vi "speed control setting.vi"() -> ()   [LabVIEW 2019]
uses:
  database.lvlib
panel:
  in  "bias 6":dbl=14.0
  in  "bias 5":dbl=14.0
  in  "bias 4":dbl=6.0
  in  "bias 3":dbl=2.0
  in  "bias 2":dbl=6.0
  in  "bias 1":dbl=12.0 caption="Set Point"
  in  "Disc 06":dbl=12.0 min=11.0 max=13.0 step=0.1
  in  "Error in 2":errorcluster
  out "Error out":errorcluster
  in  "Error THR":dbl=1.5 caption="Max. Speed (RPM)" min=0.5 max=3.0 step=0.25
  in  "Close":bool
  in  "Max. Speed (RPM)":dbl=7.5 min=5.0 max=6.0 step=0.1
  in  "Min. Speed (RPM)":dbl=5.5 min=3.0 max=4.0 step=0.1
  in  "pulse period (sec)":dbl=240.0 caption="Speed Control" min=60.0 max=600.0
  in  "Disc 05":dbl=12.0 min=11.0 max=13.0 step=0.1
  in  "Disc 04":dbl=12.0 min=11.0 max=13.0 step=0.1
  in  "Disc 03":dbl=12.0 min=11.0 max=13.0 step=0.1
  in  "Disc 02":dbl=12.0 min=11.0 max=13.0 step=0.1
  in  "Disc 01":dbl=12.0 caption="Set Point" min=10.0 max=13.0 step=0.1
  out "Name":string="Control Setting"
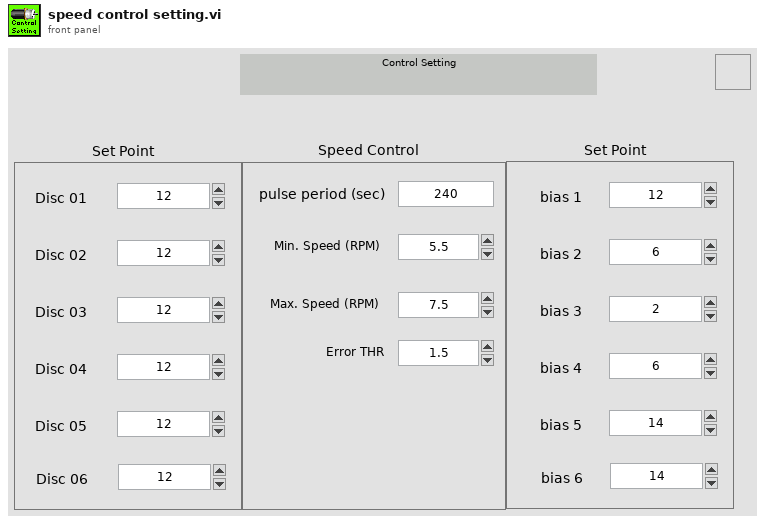
[diagram p1: front panel]
types:
  T1 = cluster{"Disc 01":dbl, "Disc 02":dbl, "Disc 03":dbl, "Disc 04":dbl, "Disc 05":dbl, "Disc 06":dbl, "pulse period (sec)":dbl, "Max. Speed (RPM)":dbl, "Min. Speed (RPM)":dbl, "Error THR":dbl, "bias 1":dbl, "bias 2":dbl, "bias 3":dbl, "bias 4":dbl, "bias 5":dbl, "bias 6":dbl}
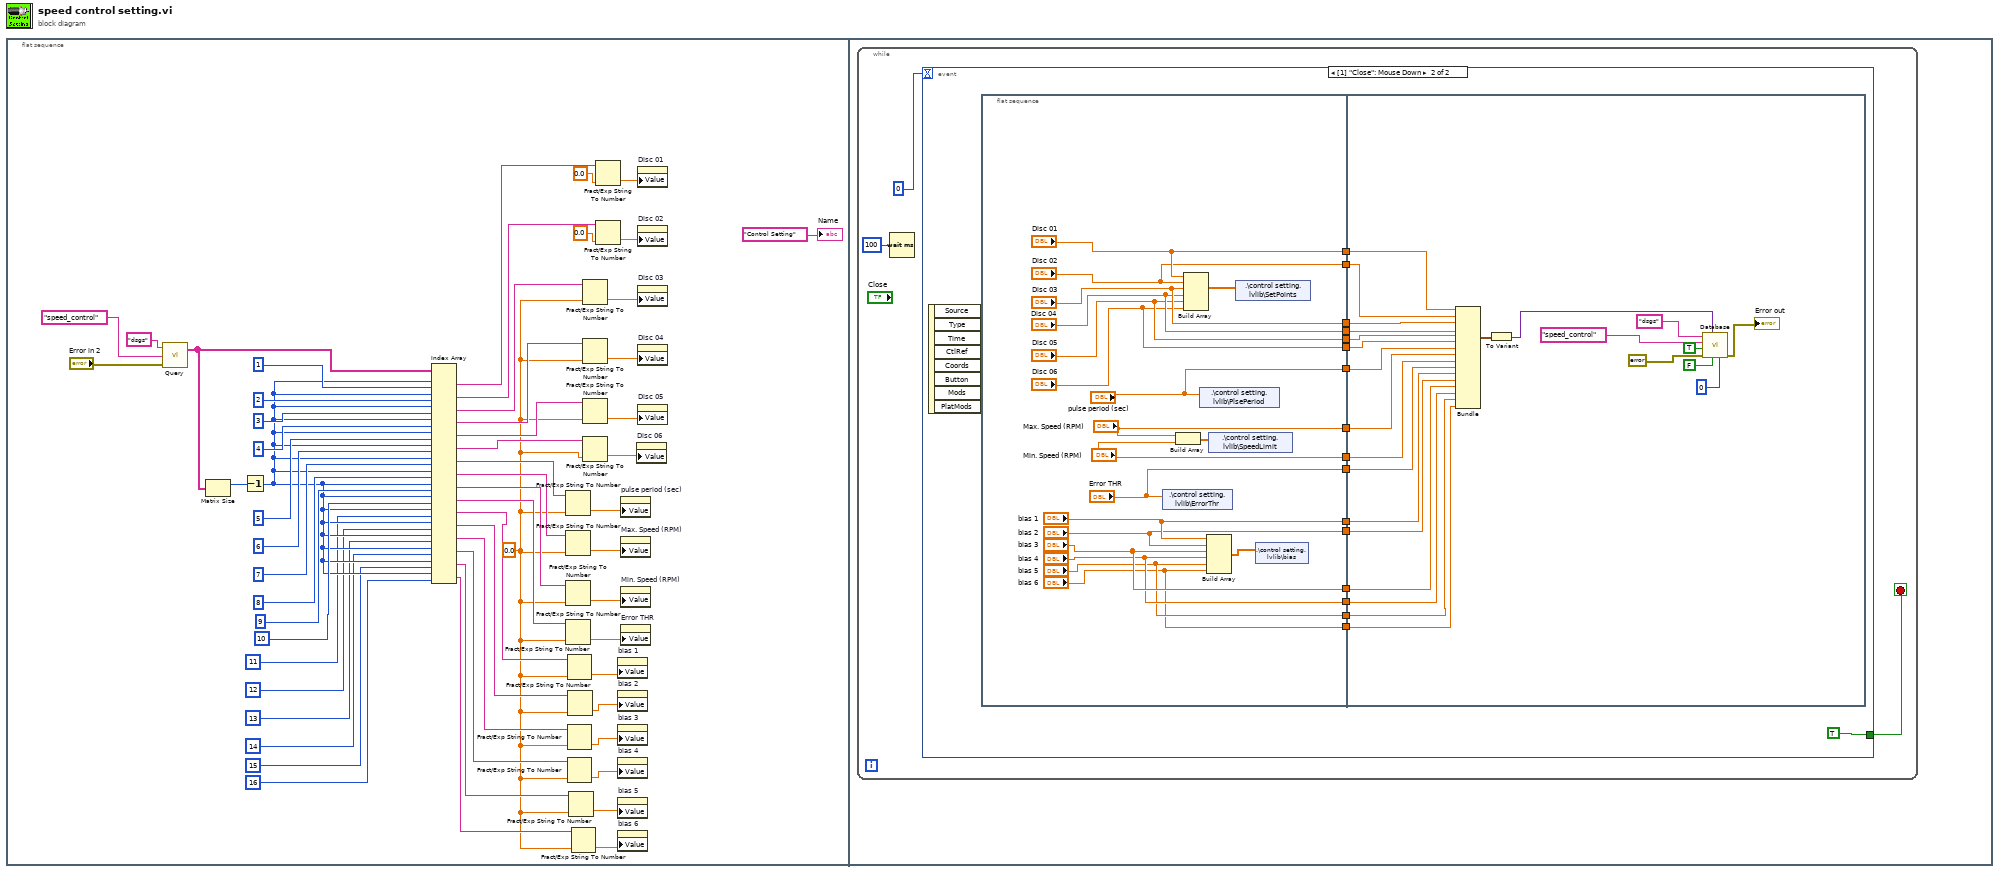
[diagram p0: block diagram]
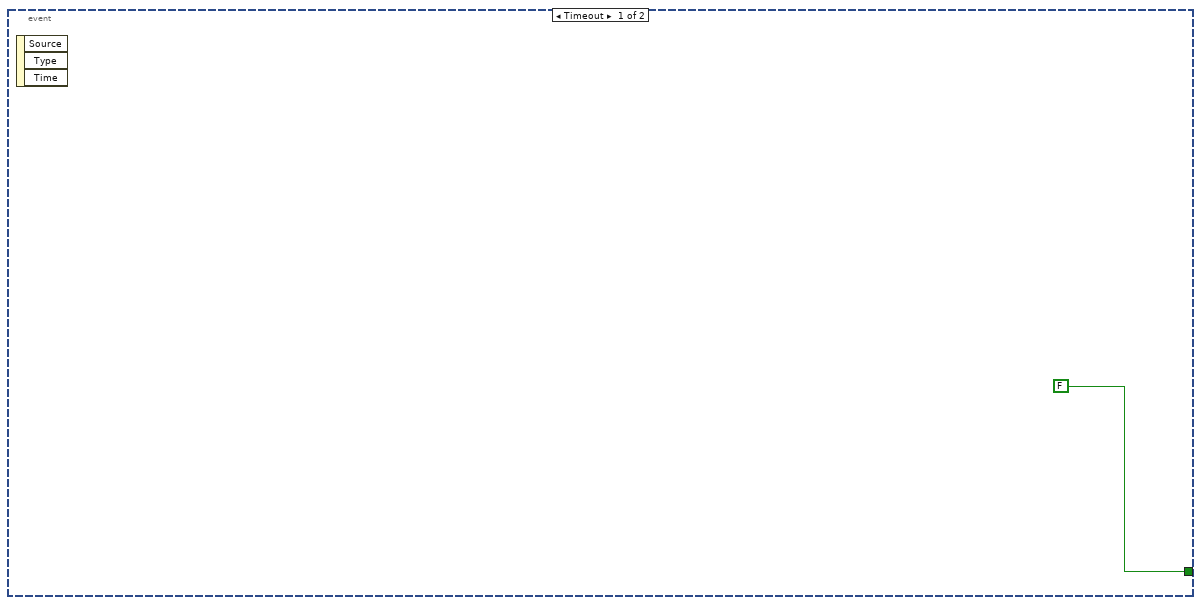
[diagram p2: hidden frame]
diagram:
  n1 = flat-sequence {
    frame #0 {
      w7 = 0.0 ("default (0 DBL)")
      n2 = call "Query.vi"("Error in"="Error in 2", "Table Name"="speed_control", "Connection Name"="dsgs") -> ("data"=w36:string[][])  [unwired: 1 in, 1 out]
      n3 = Matrix Size(0:w36) -> (1:w54:i32)  [unwired: 1 out]
      n4 = Decrement(x=w54) -> (x-1=w19:i32)
      n5 = Index Array(array=w36, index (row) #1=w19, index (col) #1=1 ("disabled index (col)"), index (row) #2=w19, index (col) #2=2 ("disabled index (col)"), index (row) #3=w19, index (col) #3=3 ("disabled index (col)"), index (row) #4=w19, index (col) #4=4 ("disabled index (col)"), index (row) #5=w19, index (col) #5=5 ("disabled index (col)"), index (row) #6=w19, index (col) #6=6 ("disabled index (col)"), index (row) #7=w19, index (col) #7=7 ("disabled index (col)"), index (row) #8=w19, index (col) #8=8 ("disabled index (col)"), index (row) #9=w19, index (col) #9=9 ("disabled index (col)"), index (row) #10=w19, index (col) #10=10 ("disabled index (col)"), index (row) #11=w19, index (col) #11=11 ("disabled index (col)"), index (row) #12=w19, index (col) #12=12 ("disabled index (col)"), index (row) #13=w19, index (col) #13=13 ("disabled index (col)"), index (row) #14=w19, index (col) #14=14 ("disabled index (col)"), index (row) #15=w19, index (col) #15=15 ("disabled index (col)"), index (row) #16=w19, index (col) #16=16 ("disabled index (col)")) -> (element #1=w44:string, element #2=w40:string, element #3=w39:string, element #4=w38:string, element #5=w37:string, element #6=w23:string, element #7=w24:string, element #8=w25:string, element #9=w26:string, element #10=w27:string, element #11=w20:string, element #12=w12:string, element #13=w11:string, element #14=w10:string, element #15=w9:string, element #16=w8:string)
      n6 = Fract/Exp String To Number(string=w24, default (0 dbl)=w7) -> (number=w31:dbl)  [unwired: 2 in, 1 out]
      n7 = Fract/Exp String To Number(string=w25, default (0 dbl)=w7) -> (number=w30:dbl)  [unwired: 2 in, 1 out]
      n8 = Fract/Exp String To Number(string=w26, default (0 dbl)=w7) -> (number=w29:dbl)  [unwired: 2 in, 1 out]
      n9 = Fract/Exp String To Number(string=w27, default (0 dbl)=w7) -> (number=w28:dbl)  [unwired: 2 in, 1 out]
      n10 = Fract/Exp String To Number(string=w20, default (0 dbl)=w7) -> (number=w6:dbl)  [unwired: 2 in, 1 out]
      n11 = Fract/Exp String To Number(string=w11, default (0 dbl)=w7) -> (number=w4:dbl)  [unwired: 2 in, 1 out]
      n12 = Fract/Exp String To Number(string=w10, default (0 dbl)=w7) -> (number=w3:dbl)  [unwired: 2 in, 1 out]
      n13 = Fract/Exp String To Number(string=w12, default (0 dbl)=w7) -> (number=w5:dbl)  [unwired: 2 in, 1 out]
      n14 = Fract/Exp String To Number(string=w9, default (0 dbl)=w7) -> (number=w2:dbl)  [unwired: 2 in, 1 out]
      n15 = Fract/Exp String To Number(string=w8, default (0 dbl)=w7) -> (number=w1:dbl)  [unwired: 2 in, 1 out]
      n16 = Fract/Exp String To Number(string=w39, default (0 dbl)=w7) -> (number=w34:dbl)  [unwired: 2 in, 1 out]
      n17 = Fract/Exp String To Number(string=w38, default (0 dbl)=w7) -> (number=w33:dbl)  [unwired: 2 in, 1 out]
      n18 = Fract/Exp String To Number(string=w37, default (0 dbl)=w7) -> (number=w32:dbl)  [unwired: 2 in, 1 out]
      n19 = Fract/Exp String To Number(string=w23, default (0 dbl)=w7) -> (number=w22:dbl)  [unwired: 2 in, 1 out]
      n20 = Fract/Exp String To Number(string=w44, default (0 dbl)=0.0 ("default (0 DBL)")) -> (number=w42:dbl)  [unwired: 2 in, 1 out]
      n21 = Fract/Exp String To Number(string=w40, default (0 dbl)=0.0 ("default (0 DBL)")) -> (number=w35:dbl)  [unwired: 2 in, 1 out]
      n22 = property on="bias 1" class="DigNum (strict)"("Value"=w6) -> ()  [unwired: 2 in, 2 out]
      n23 = property on="bias 2" class="DigNum (strict)"("Value"=w5) -> ()  [unwired: 2 in, 2 out]
      n24 = property on="bias 3" class="DigNum (strict)"("Value"=w4) -> ()  [unwired: 2 in, 2 out]
      n25 = property on="bias 4" class="DigNum (strict)"("Value"=w3) -> ()  [unwired: 2 in, 2 out]
      n26 = property on="bias 5" class="DigNum (strict)"("Value"=w2) -> ()  [unwired: 2 in, 2 out]
      n27 = property on="bias 6" class="DigNum (strict)"("Value"=w1) -> ()  [unwired: 2 in, 2 out]
      n28 = property on="pulse period (sec)" class="DigNum (strict)"("Value"=w31) -> ()  [unwired: 2 in, 2 out]
      n29 = property on="Max. Speed (RPM)" class="DigNum (strict)"("Value"=w30) -> ()  [unwired: 2 in, 2 out]
      n30 = property on="Min. Speed (RPM)" class="DigNum (strict)"("Value"=w29) -> ()  [unwired: 2 in, 2 out]
      n31 = property on="Error THR" class="DigNum (strict)"("Value"=w28) -> ()  [unwired: 2 in, 2 out]
      n32 = property on="Disc 06" class="DigNum (strict)"("Value"=w22) -> ()  [unwired: 2 in, 2 out]
      n33 = property on="Disc 01" class="DigNum (strict)"("Value"=w42) -> ()  [unwired: 2 in, 2 out]
      n34 = property on="Disc 02" class="DigNum (strict)"("Value"=w35) -> ()  [unwired: 2 in, 2 out]
      n35 = property on="Disc 03" class="DigNum (strict)"("Value"=w34) -> ()  [unwired: 2 in, 2 out]
      n36 = property on="Disc 04" class="DigNum (strict)"("Value"=w33) -> ()  [unwired: 2 in, 2 out]
      n37 = property on="Disc 05" class="DigNum (strict)"("Value"=w32) -> ()  [unwired: 2 in, 2 out]
      "Name" <- "Control Setting" ("Name")
    }
    frame #1 {
      n38 = while {
        stop <- w60 stop-if-true
        n39 = Wait (ms)(milliseconds to wait=u32 100) -> ()  [unwired: 1 out]
        n40 = event shown="[1] \"Close\": Mouse Down" {
          selector: _ -> [_ _]
          dyn-events: _ -> [_ _]
          timeout: 0 -> [_ _]
          tunnel: [FALSE TRUE] -> w60
          event Timeout {
            n41 = event-data() -> ()  [unwired: 1 in, 3 out]
          }
          event "Close": Mouse Down {
            n42 = event-data() -> ()  [unwired: 1 in, 8 out]
            n43 = flat-sequence {
              tunnel: ["Disc 01"] -> w78
              tunnel: ["Disc 02"] -> w77
              tunnel: ["Disc 03"] -> w76
              tunnel: ["Disc 04"] -> w75
              tunnel: ["Disc 05"] -> w74
              tunnel: ["pulse period (sec)"] -> w73
              tunnel: ["Max. Speed (RPM)"] -> w72
              tunnel: ["Min. Speed (RPM)"] -> w71
              tunnel: ["Error THR"] -> w70
              tunnel: ["Disc 06"] -> w69
              tunnel: ["bias 1"] -> w68
              tunnel: ["bias 2"] -> w67
              tunnel: ["bias 3"] -> w66
              tunnel: ["bias 4"] -> w65
              tunnel: ["bias 5"] -> w64
              tunnel: ["bias 6"] -> w63
              tunnel: w78 -> [w121]
              tunnel: w77 -> [w120]
              tunnel: w76 -> [w119]
              tunnel: w75 -> [w118]
              tunnel: w74 -> [w117]
              tunnel: w73 -> [w106]
              tunnel: w72 -> [w107]
              tunnel: w71 -> [w108]
              tunnel: w70 -> [w109]
              tunnel: w69 -> [w105]
              tunnel: w68 -> [w104]
              tunnel: w67 -> [w103]
              tunnel: w66 -> [w102]
              tunnel: w65 -> [w101]
              tunnel: w64 -> [w100]
              tunnel: w63 -> [w99]
              frame #0 {
                n44 = shared-variable ".\\control setting.lvlib\\ErrorThr"("Error THR") -> ()  [unwired: 1 in, 1 out]
                n45 = Build Array("Max. Speed (RPM)", "Min. Speed (RPM)") -> (w97:dbl[])
                n46 = Build Array("Disc 01", "Disc 02", "Disc 03", "Disc 04", "Disc 05", "Disc 06") -> (w98:dbl[])
                n47 = shared-variable ".\\control setting.lvlib\\PlsePeriod"("pulse period (sec)") -> ()  [unwired: 1 in, 1 out]
                n48 = Build Array("bias 1", "bias 2", "bias 3", "bias 4", "bias 5", "bias 6") -> (w86:dbl[])
                n49 = shared-variable ".\\control setting.lvlib\\SpeedLimit"(w97) -> ()  [unwired: 1 in, 1 out]
                n50 = shared-variable ".\\control setting.lvlib\\SetPoints"(w98) -> ()  [unwired: 1 in, 1 out]
                n51 = shared-variable ".\\control setting.lvlib\\bias"(w86) -> ()  [unwired: 1 in, 1 out]
              }
              frame #1 {
                n52 = Bundle("Disc 01"=w121, "Disc 02"=w120, "Disc 03"=w119, "Disc 04"=w118, "Disc 05"=w117, "Disc 06"=w105, "pulse period (sec)"=w106, "Max. Speed (RPM)"=w107, "Min. Speed (RPM)"=w108, "Error THR"=w109, "bias 1"=w104, "bias 2"=w103, "bias 3"=w102, "bias 4"=w101, "bias 5"=w100, "bias 6"=w99) -> (w116:T1)  [unwired: 1 in]
                n53 = To Variant(anything=w116) -> (Variant=w115:variant)
                n54 = call "Database.vi"("Maximum Row"=0, "Delete row?"=FALSE, "Data"=w115, "Error in"=errorcluster {"status"=FALSE, "code"=0, "source"=""}, "Auto Increment ID?"=TRUE, "Table"="speed_control", "Connection"="dsgs") -> ("Error out"=→"Error out":errorcluster)  [unwired: 4 in]
              }
            }
          }
        }
      }
    }
  }
